vi "mono_step.vi"(7 "Steering Wheel Angle":dbl(knob) scale=-1.0..1.0, 8 "error_in":errorcluster, 9 "Throttle":dbl(slide) scale=-1.0..1.0, 10 "Python Module Path":path, 11 "Refnum in":refnum<k35>) -> (0 "error_out":errorcluster, 1 "Waveform Chart":dbl(graph), 2 "Speed":dbl(knob) scale=0.0..200.0, 3 "Refnum out":refnum<k35>, 4 "return value":i32[](array[numeric]))   [LabVIEW 2018]
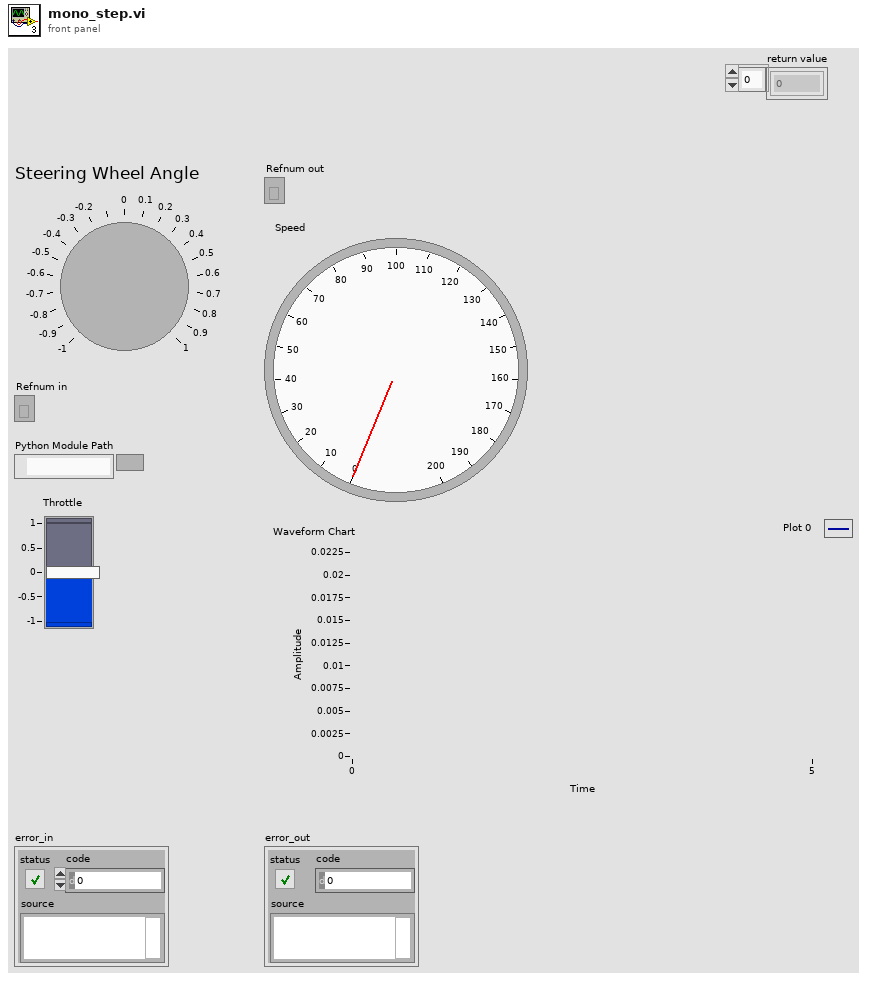
[diagram p1: front panel]
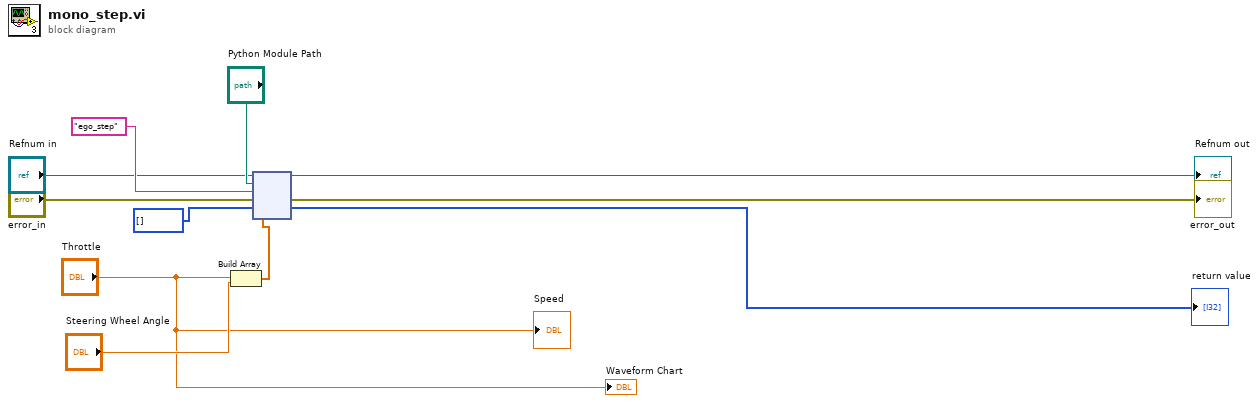
[diagram p0: block diagram]
diagram:
  n1 = Build Array("Throttle", "Steering Wheel Angle") -> (w6:dbl[])
  n2 = node("Refnum in", "Python Module Path", "ego_step" ("function name"), "error_in", i32[] [], w6) -> (→"Refnum out":refnum<k35>, →"error_out":errorcluster, →"return value":i32[])  [unwired: 1 in, 2 out]
  "Speed" <- "Throttle"
  "Waveform Chart" <- "Throttle"
